vi "Arrange VIWin - Ensure Leftmost BD Object Is Visible.vi"(0 "VI in":refnum<vi>, 1 "BD canvas margin":i16, 11 "error in":errorcluster) -> (15 "error out":errorcluster)   [LabVIEW 2017, in "Arrange VI Window.lvlib"]
uses:
  Arrange VI Window.lvlib
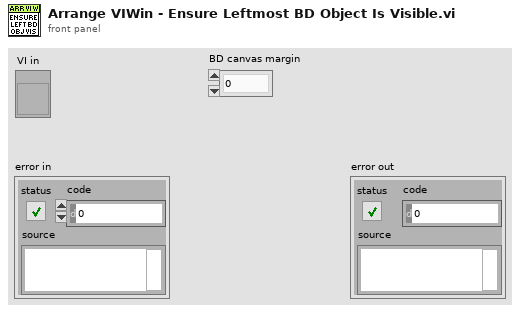
[diagram p1: front panel]
types:
  T1 = typedef "LVBoundsTypeDef.ctl" = cluster{"Width":u32, "Height":u32}
  T2 = typedef "LVRectTypeDef.ctl" = cluster{"Left":i16, "Top":i16, "Right":i16, "Bottom":i16}
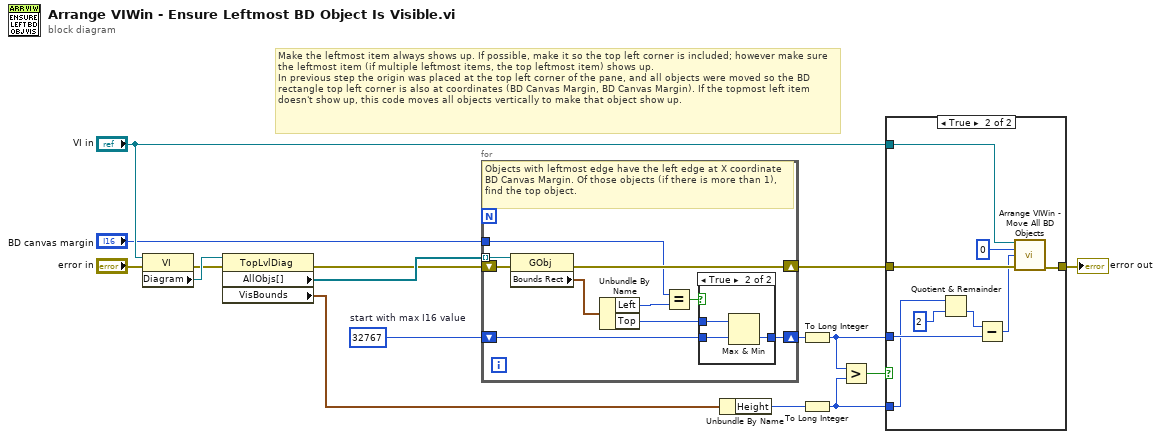
[diagram p0: block diagram]
diagram:
  w8 = i16 32767  # start with max I16 value
  # "Make the leftmost item always shows up. If possible, make it so the top left corner is included; however make sure the leftmost item (if multiple leftmost items, the top leftmost item) shows up.\nIn previous step the origin was placed at the top left corner of the pane, and all objects were moved so the BD rectangle top left corner is also at coordinates (BD Canvas Margin, BD Canvas Margin). If the topmost left item doesn't show up, this code moves all objects vertically to make that object show up."
  n1 = property on="Property Node" class="VI"(reference="VI in", error in="error in") -> (error out=w15:errorcluster, "Diagram"=w16:refnum<vi>)  [unwired: 1 out]
  n2 = property on="Property Node" class="TopLvlDiag"(reference=w16, error in=w15) -> (error out=w2:errorcluster, "AllObjs[]"=w9:refnum<vi>[], "VisBounds"=w11:T1)  [unwired: 1 out]
  n3 = for {
    shift-right: [w24] -> w10
    shift-left: w2 -> [w26]
    shift-right: [w23] -> w4
    shift-left: w8 -> [w22]
    tunnel: w9 -> [w21] mode=indexing
    tunnel: "BD canvas margin" -> [w17]
    # "Objects with leftmost edge have the left edge at X coordinate BD Canvas Margin. Of those objects (if there is more than 1), find the top object."
    n4 = property on="Property Node" class="GObj"(reference=w21, error in=w26) -> (error out=w24:errorcluster, "Bounds Rect"=w25:T2)  [unwired: 1 out]
    n5 = Unbundle By Name(w25) -> ("Left"=w19:i16, "Top"=w20:i16)
    n6 = Equal?(x=w17, y=w19) -> (x = y?=w18:bool)
    n7 = case shown="True" w18 {
      tunnel: [w27 w30] -> w23
      tunnel: w22 -> [w27 w29]
      tunnel: w20 -> [_ w28]
      frame False {
      }
      frame True {
        n8 = Max & Min(x=w28, y=w29) -> (min(x,y)=w30:i16)  [unwired: 1 out]
      }
    }
  }
  n9 = Unbundle By Name(w11) -> ("Height"=w12:u32)
  n10 = To Long Integer(number=w4) -> (32bit integer=w1:i32)
  n11 = To Long Integer(number=w12) -> (32bit integer=w5:i32)
  n12 = Greater?(x=w1, y=w5) -> (0:w6:bool)
  n13 = case shown="True" w6 {
    tunnel: w10 -> [w31 w36]
    tunnel: [w31 w37] -> w7
    tunnel: "VI in" -> [_ w35]
    tunnel: w1 -> [_ w39]
    tunnel: w5 -> [_ w38]
    frame False {
    }
    frame True {
      n14 = Quotient & Remainder(x=w38, y=2) -> (floor(x/y)=w33:i32)  [unwired: 1 out]
      n15 = Subtract(x=w33, y=w39) -> (x-y=w32:i32)
      n16 = call "Arrange VIWin - Move All BD Objects.vi"("VI in"=w35, "x delta"=0, "y delta"=w32, "error in"=w36) -> ("error out"=w37:errorcluster)  [unwired: 11 in]
    }
  }
  "error out" <- w7
